vi "Convert Database Datatype.vi"(1 "ADODB data type":T2) -> (0 "Database data type":T1=enum."String")   [LabVIEW 2020, in "ADODB.lvlib"]
uses:
  ADODB.lvlib
  <vilib>/addons/database/Auxilliary.llb/DB Tools DataTypes.ctl
  Database Interfaces/Database data type.ctl
  Database Interfaces.lvlib
  <vilib>/addons/database/NI_Database_API.lvlib
panel:
  # "Use this VI to convert between ADODB (database connectivity toolkit) data types to Database Interface data types"
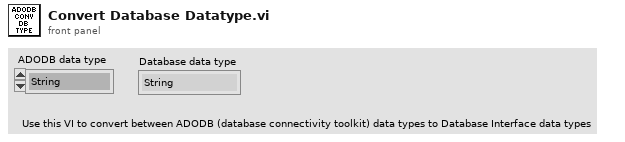
[diagram p1: front panel]
types:
  T1 = typedef "Database Interfaces.lvlib/Database data type.ctl" = enum16{"Undefined", "String", "Long (I32)", "Single (SGL)", "Double (DBL)", "Date/Time", "Binary"}
  T2 = typedef "NI_Database_API.lvlib/DB Tools DataTypes.ctl" = enum16{"String", "Long (I32)", "Single (SGL)", "Double (DBL)", "Date/Time", "Binary"}
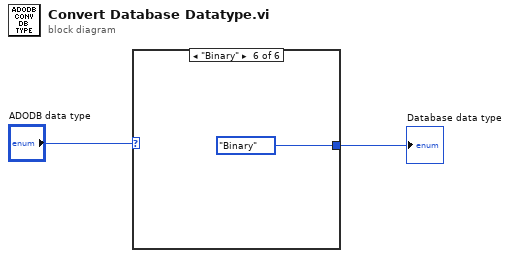
[diagram p0: block diagram]
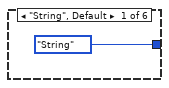
[diagram p2: hidden frame]
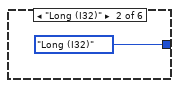
[diagram p3: hidden frame]
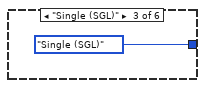
[diagram p4: hidden frame]
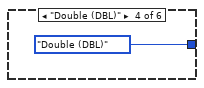
[diagram p5: hidden frame]
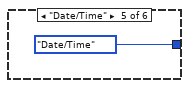
[diagram p6: hidden frame]
diagram:
  n1 = case shown="\"Binary\"" "ADODB data type" {
    tunnel: [Database_data_type."String" ("Database data type") Database_data_type."Long (I32)" ("Database data type") Database_data_type."Single (SGL)" ("Database data type") Database_data_type."Double (DBL)" ("Database data type") Database_data_type."Date/Time" ("Database data type") Database_data_type."Binary" ("Database data type")] -> w1
    frame "String", Default {
    }
    frame "Long (I32)" {
    }
    frame "Single (SGL)" {
    }
    frame "Double (DBL)" {
    }
    frame "Date/Time" {
    }
    frame "Binary" {
    }
  }
  "Database data type" <- w1
